vi "XIPIN_Video_over_IP_FEC_Receiver_1_0.vi"   [LabVIEW 2017]
doc: "The Xilinx, Inc LogiCORE IP Video over IP FEC Receiver is a broadcast application module that recovers lost packets from RTP encapsulated payloads using SMPTE 2022 Forward Error Correction method. It is capable of handling a large number of video streams and is suited for deploying in 1 Gb/s networks\n------------------------------------\n<b>Need License</b> : Yes\n<b>Interface</b> : AXI4 AXI4-Stream"
uses:
  <vilib>/rvi/XilinxIP/XIPIN_XNode/niFpgaXIPIN.xnode
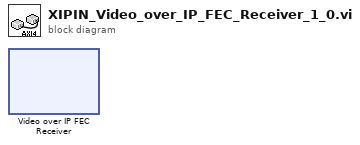
[diagram p0: block diagram]
diagram:
  n1 = xnode ("Video over IP FEC Receiver")() -> ()
